vi "6733_voltage_conversions.vi"(9 "Final Value":dbl, 10 "Initial value":dbl, 11 "Conversion":T1) -> (1 "Final Voltage":dbl, 2 "Initial voltage":dbl)   [LabVIEW 2015]
uses:
  6733_voltage_conversions.ctl
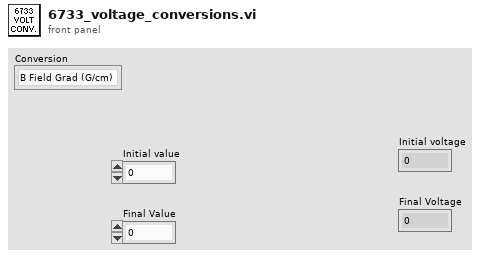
[diagram p1: front panel]
types:
  T1 = typedef "6733_voltage_conversions.ctl" = enum16{"B Field Grad (G/cm)", "Red AOM Center Freq (MHz)", "Red Dither Pk(kHz)", "Red Power (mW)", "Volts"}
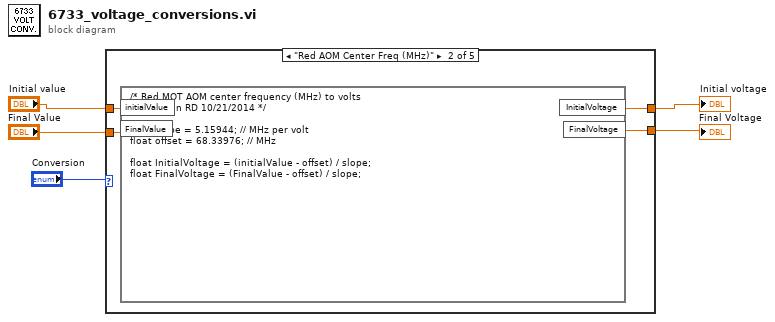
[diagram p0: block diagram]
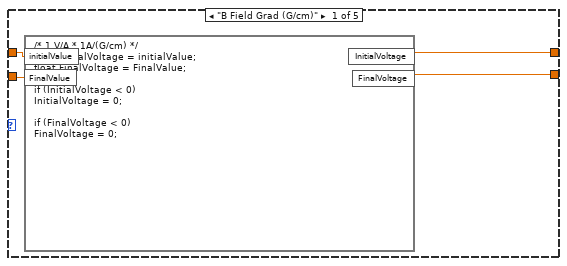
[diagram p2: hidden frame]
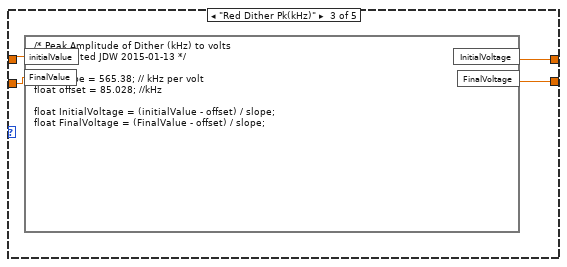
[diagram p3: hidden frame]
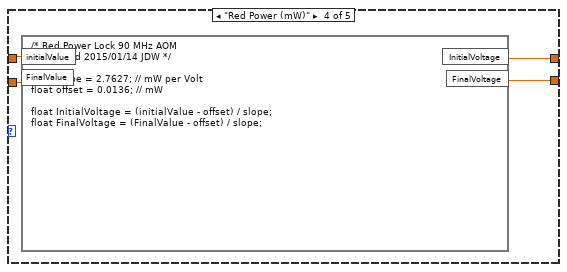
[diagram p4: hidden frame]
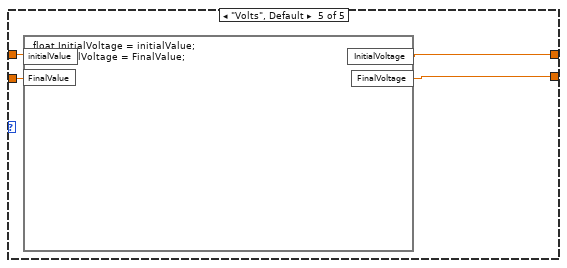
[diagram p5: hidden frame]
diagram:
  n1 = case shown="\"Red AOM Center Freq (MHz)\"" "Conversion" {
    tunnel: "Initial value" -> [w6 w13 w14 w21 w23]
    tunnel: "Final Value" -> [w7 w12 w15 w20 w22]
    tunnel: [w9 w11 w16 w18 w24] -> w2
    tunnel: [w8 w10 w17 w19 w25] -> w1
    frame "B Field Grad (G/cm)" {
      n2 = formula code="/* 1 V/A * 1A/(G/cm) */\nfloat InitialVoltage = initialValue;\nfloat FinalVoltage = FinalValue;\n\nif (InitialVoltage < 0)\nInitialVoltage = 0;\n\nif (FinalVoltage < 0)\nFinalVoltage = 0;"("initialValue"=w6, "FinalValue"=w7) -> ("InitialVoltage"=w9:dbl, "FinalVoltage"=w8:dbl)
    }
    frame "Red AOM Center Freq (MHz)" {
      n3 = formula code="/* Red MOT AOM center frequency (MHz) to volts\ncalibration RD 10/21/2014 */\n\nfloat slope = 5.15944; // MHz per volt\nfloat offset = 68.33976; // MHz\n\nfloat InitialVoltage = (initialValue - offset) / slope;\nfloat FinalVoltage = (FinalValue - offset) / slope;"("initialValue"=w13, "FinalValue"=w12) -> ("InitialVoltage"=w11:dbl, "FinalVoltage"=w10:dbl)
    }
    frame "Red Dither Pk(kHz)" {
      n4 = formula code="/* Peak Amplitude of Dither (kHz) to volts\n    Calibrated JDW 2015-01-13 */\n\nfloat slope = 565.38; // kHz per volt\nfloat offset = 85.028; //kHz\n\nfloat InitialVoltage = (initialValue - offset) / slope;\nfloat FinalVoltage = (FinalValue - offset) / slope;"("initialValue"=w14, "FinalValue"=w15) -> ("InitialVoltage"=w16:dbl, "FinalVoltage"=w17:dbl)
    }
    frame "Red Power (mW)" {
      n5 = formula code="/* Red Power Lock 90 MHz AOM\nCalibrated 2015/01/14 JDW */\n\nfloat slope = 2.7627; // mW per Volt\nfloat offset = 0.0136; // mW\n\nfloat InitialVoltage = (initialValue - offset) / slope;\nfloat FinalVoltage = (FinalValue - offset) / slope;"("initialValue"=w21, "FinalValue"=w20) -> ("InitialVoltage"=w18:dbl, "FinalVoltage"=w19:dbl)
    }
    frame "Volts", Default {
      n6 = formula code="float InitialVoltage = initialValue;\nfloat FinalVoltage = FinalValue;"("initialValue"=w23, "FinalValue"=w22) -> ("InitialVoltage"=w24:dbl, "FinalVoltage"=w25:dbl)
    }
  }
  "Initial voltage" <- w2
  "Final Voltage" <- w1
